vi "Lift Master Master.vi"(0 "left output range":cluster{"output high":dbl, "output low":dbl}={"output high"=100.0, "output low"=-100.0} {"output low" format="%.2f"; "output high" format="%.2f"}, 1 "reset max":bool, 2 "left encoder":dbl, 5 "right output range":cluster{"output high":dbl, "output low":dbl}={"output high"=100.0, "output low"=-100.0} {"output low" format="%.2f"; "output high" format="%.2f"}, 7 "move to distance":dbl, 9 "left PID gains":T1={"proportional gain (Kc)"=1.0, "integral time (Ti, min)"=0.01, "derivative time (Td, min)"=0.0} {"derivative time (Td, min)" format="%.3f"; "integral time (Ti, min)" format="%.3f"; "proportional gain (Kc)" format="%.3f"}, 11 "right PID gains":T1={"proportional gain (Kc)"=1.0, "integral time (Ti, min)"=0.01, "derivative time (Td, min)"=0.0} {"derivative time (Td, min)" format="%.3f"; "integral time (Ti, min)" format="%.3f"; "proportional gain (Kc)" format="%.3f"}, 12 "move to":bool, 13 "right encoder":dbl) -> (4 "lift motor left":dbl=-0.25, 6 "lift motor right":dbl=0.5, 8 "max difference":dbl, 10 "encoder count left":dbl, 14 "left to target difference":dbl, 15 "encoder count right":dbl)   [LabVIEW 2014]
uses:
  <vilib>/addons/control/pid/pid.llb/PID (DBL).vi
  <vilib>/addons/control/pid/NI_PID_pid.lvlib
panel:
  in  "last max difference":dbl
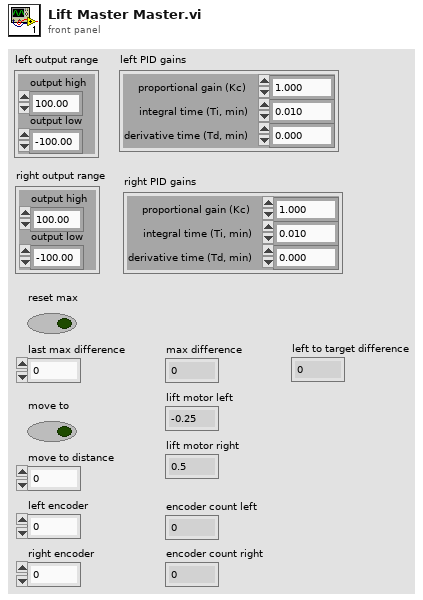
[diagram p1: front panel]
types:
  T1 = cluster{"proportional gain (Kc)":dbl, "integral time (Ti, min)":dbl, "derivative time (Td, min)":dbl}
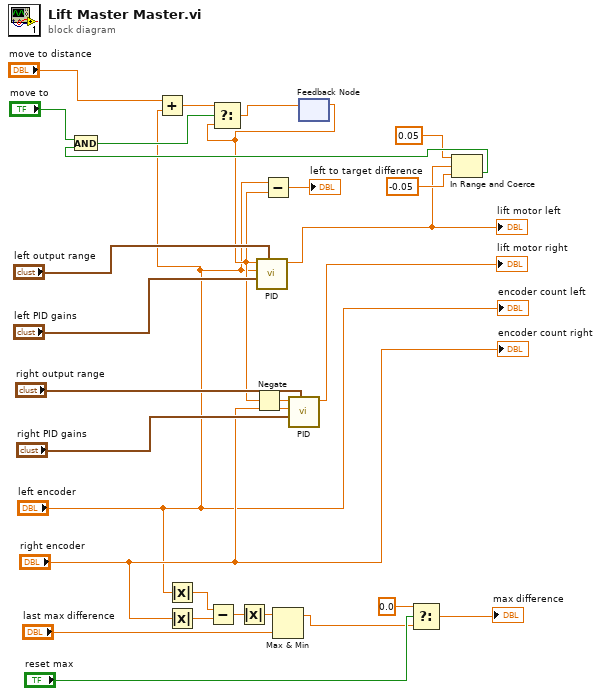
[diagram p0: block diagram]
diagram:
  n1 = Add(x="move to distance", y="left encoder") -> (x+y=w23:dbl)
  n2 = Absolute Value(x="left encoder") -> (abs(x)=w11:dbl)
  n3 = Absolute Value(x="right encoder") -> (abs(x)=w12:dbl)
  n4 = Subtract(x=w11, y=w12) -> (x-y=w13:dbl)
  n5 = Absolute Value(x=w13) -> (abs(x)=w14:dbl)
  n6 = Max & Min(x=w14, y="last max difference") -> (max(x,y)=w15:dbl)  [unwired: 1 out]
  n7 = feedback #1() -> (w4:dbl)  [unwired: 1 in]
  n8 = Negate(x=w4) -> (-x=w3:dbl)
  n9 = call-poly <vilib>:"PID.vi"("output range"="left output range", "PID gains"="left PID gains", "process variable"="left encoder", "setpoint"=w4) -> ("output"=w19:dbl)  [unwired: 6 in, 1 out]
  "lift motor left" <- w19
  n10 = Subtract(x="left encoder", y=w4) -> (x-y=→"left to target difference":dbl)
  n11 = call-poly <vilib>:"PID.vi"("output range"="right output range", "PID gains"="right PID gains", "process variable"="right encoder", "setpoint"=w3) -> ("output"=→"lift motor right":dbl)  [unwired: 6 in, 1 out]
  n12 = Select(t=0.0, s="reset max", f=w15) -> (s? t:f=→"max difference":dbl)
  n13 = In Range and Coerce(upper limit=0.05, x=w19, lower limit=-0.05) -> (In Range?=w22:bool)  [unwired: 1 out]
  n14 = And(x="move to", y=w22) -> (x .and. y?=w25:bool)
  n15 = Select(t=w23, s=w25, f=w4) -> (s? t:f=w24:dbl)
  n16 = feedback-in #1(w24) -> ()
  "encoder count left" <- "left encoder"
  "encoder count right" <- "right encoder"
